vi "CBL Erase Flash.vi"(5 "TimeOut":u32, 6 "FlashEndAddr":u32, 7 "FlashStartAddr":u32, 9 "NodeAddr":u8, 10 "CANIndex":i32, 11 "DevIndex":i32) -> (3 "function return":i32)   [LabVIEW 2010, in "CANBootloader.lvlib"]
doc: "int WINAPI CBL_EraseFlash(int DevIndex,int CANIndex,unsigned char NodeAddr,unsigned int FlashStartAddr,unsigned int FlashEndAddr,unsigned int TimeOut);"
uses:
  CANBootloader.lvlib
  CANBootloader/Ginkgo_Driver.dll
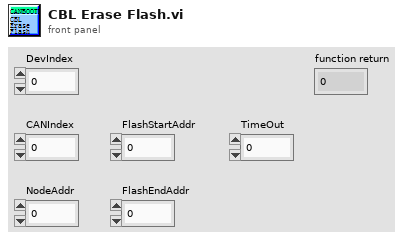
[diagram p1: front panel]
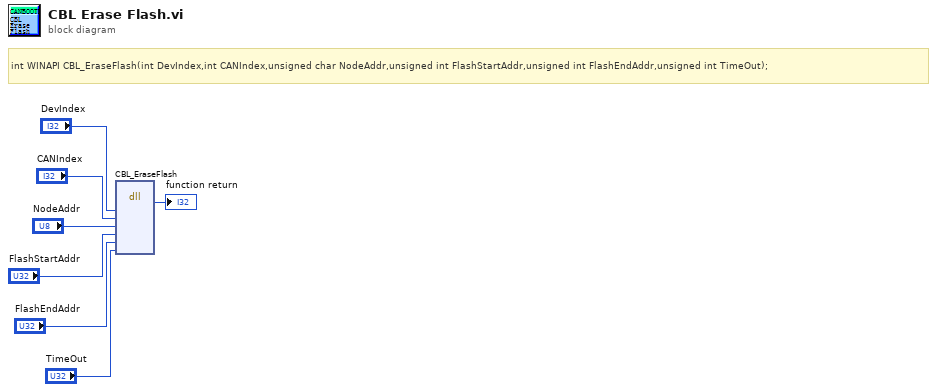
[diagram p0: block diagram]
diagram:
  # "int WINAPI CBL_EraseFlash(int DevIndex,int CANIndex,unsigned char NodeAddr,unsigned int FlashStartAddr,unsigned int FlashEndAddr,unsigned int TimeOut);"
  n1 = dll-call lib="E:/Project/vt_ginkgo/truck/Ginkgo Driver/vs2010/Ginkgo_USB-I2C&SPI&CAN_API_v2.0.3.3/lib/labview_32bit/CANBootloader/Ginkgo_Driver.*" fn="CBL_EraseFlash"("DevIndex"="DevIndex", "CANIndex"="CANIndex", "NodeAddr"="NodeAddr", "FlashStartAddr"="FlashStartAddr", "FlashEndAddr"="FlashEndAddr", "TimeOut"="TimeOut") -> (→"function return":i32)  [unwired: 9 in, 2 out]
